vi "Dakota_6Valves.vi"(3 "C/AO0":i32(knob)=472 min=0 max=1023 scale=0.0..1023.0 scale format="%.2f") -> ()   [LabVIEW 2015]
uses:
  <vilib>/rvi/Emulation/niFpgaGetClockAttributes.vi
  <vilib>/rvi/Emulation/niFpgaSctlEmulationGetInTimedLoop.vi
  <vilib>/rvi/Emulation/niFpgaEmulationReportErrorSimple.vi
  <vilib>/rvi/eio/common/nirviEmuTemplateMethod_errors.vi
  <vilib>/rvi/interface/RandomDataEmulation/niFpgaRandomDataHandleErrors.vi
  <vilib>/rvi/Emulation/niFpgaCriticalErrorInLSC.vi
  <vilib>/eio/EIONode/EIONode.xnode
  <vilib>/rvi/DataTransferAndStorage/Container/XNode/niFpgaContainer.xnode
  <vilib>/rvi/interface/RandomDataEmulation/nirviRandomDataFpgaReadWriteTemplate.vi
panel:
  in  "Inlet Count(uSec) 5":i32 caption="Count(uSec)"
  out "A/AO0 Overflow?":bool
  in  "A/AO0":i32(knob)=472 min=0 max=4095 scale=0.0..4095.0 scale format="%.2f"
  in  "Inlet Count(uSec) 4":i32 caption="Count(uSec)"
  out "A/AO1 Overflow?":bool
  in  "A/AO1":i32(knob)=472 min=0 max=4095 scale=0.0..4095.0 scale format="%.2f"
  in  "Inlet Count(uSec) 3":i32 caption="Count(uSec)"
  out "B/AO0 Overflow?":bool
  in  "B/AO0":i32(knob)=472 min=0 max=4095 scale=0.0..4095.0 scale format="%.2f"
  in  "Inlet Count(uSec) 2":i32 caption="Count(uSec)"
  out "B/AO1 Overflow?":bool
  in  "B/AO1":i32(knob)=472 min=0 max=4095 scale=0.0..4095.0 scale format="%.2f"
  in  "Outlet Count(uSec)":i32 caption="Count(uSec)"
  out "C/AO1 Overflow?":bool
  in  "C/AO1":i32(knob)=405 min=0 max=1023 scale=0.0..1023.0 scale format="%.2f"
  in  "Inlet Count(uSec)":i32 caption="Count(uSec)"
  out "C/AO0 Overflow?":bool
  # "Overview\n======\n\nThis demonstrates how to control the PSV105 Valve. At 0 bits, the voltage across the 250 ohms, 30W resistor is 1.3V. This corresponds to 5.2mA, a little above the required current to turn the valve on according to the manufacturer. At 910 bits, we obtain a voltage of 5V across the shunt resistor; this corresponds to 20mA. \n\nConnection Protocols\n===============\nWire the AO0 pin on the C connector of the myRIo to the pin 3 of the non-inverting input of the opamp. Connect the power supplies andfollow the following instructions:\n\nInstructions:\n1.        Operate at constant pressure of 30 psi to get best results\n2.        Operate this valve between the DAC resolutions of 0 and  717 only. If you operate outside of this range, you might damage the valve.\n3.        Run the VI."
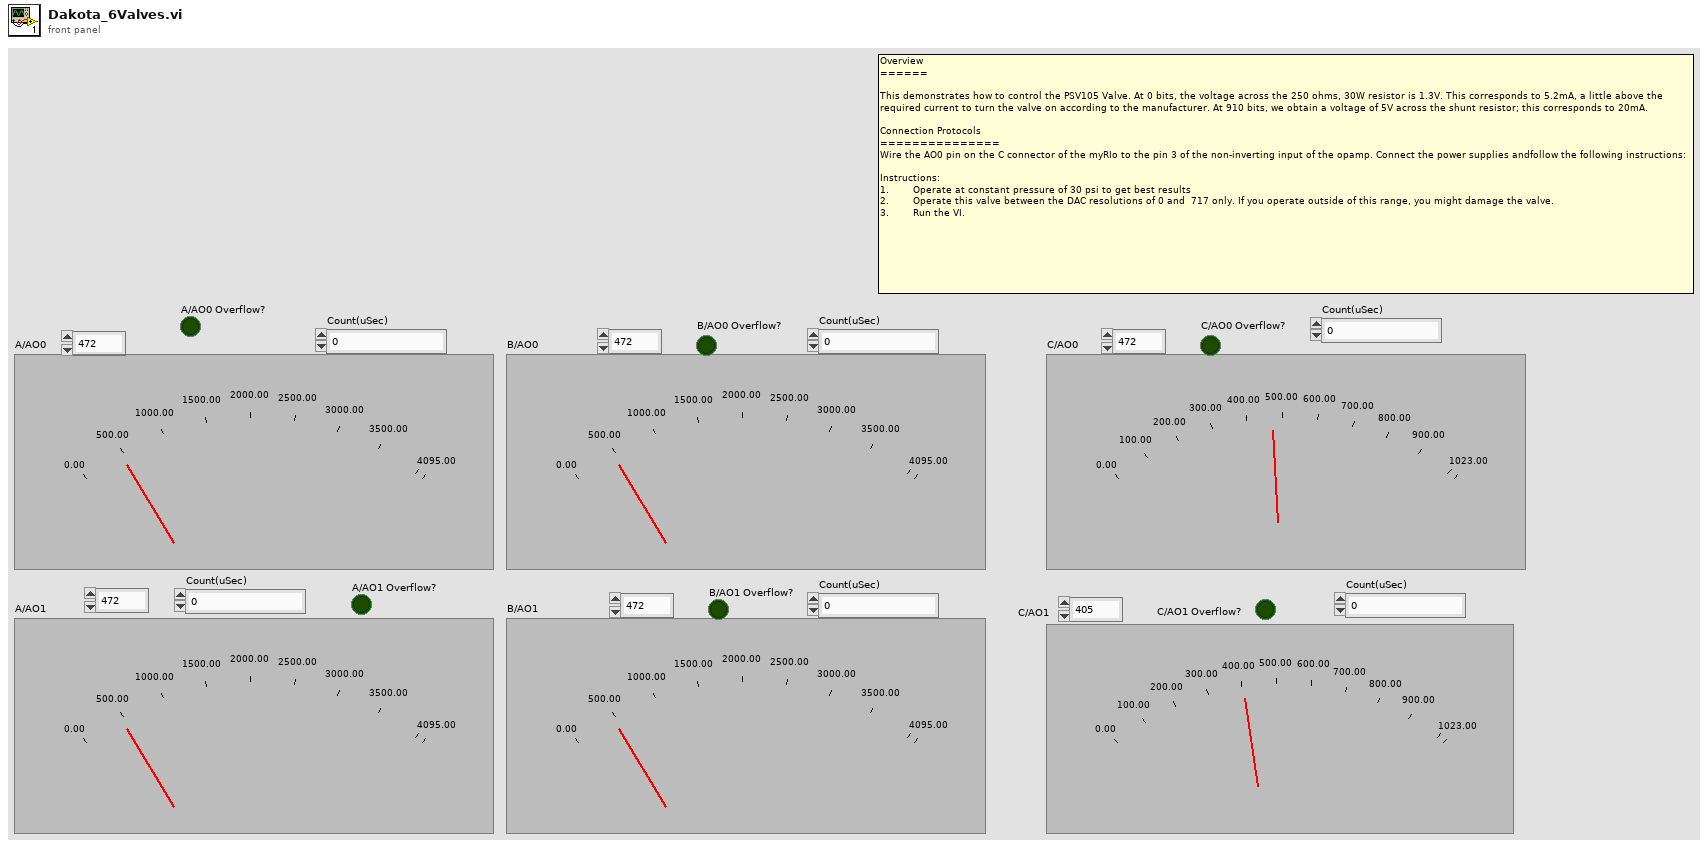
[diagram p1: front panel]
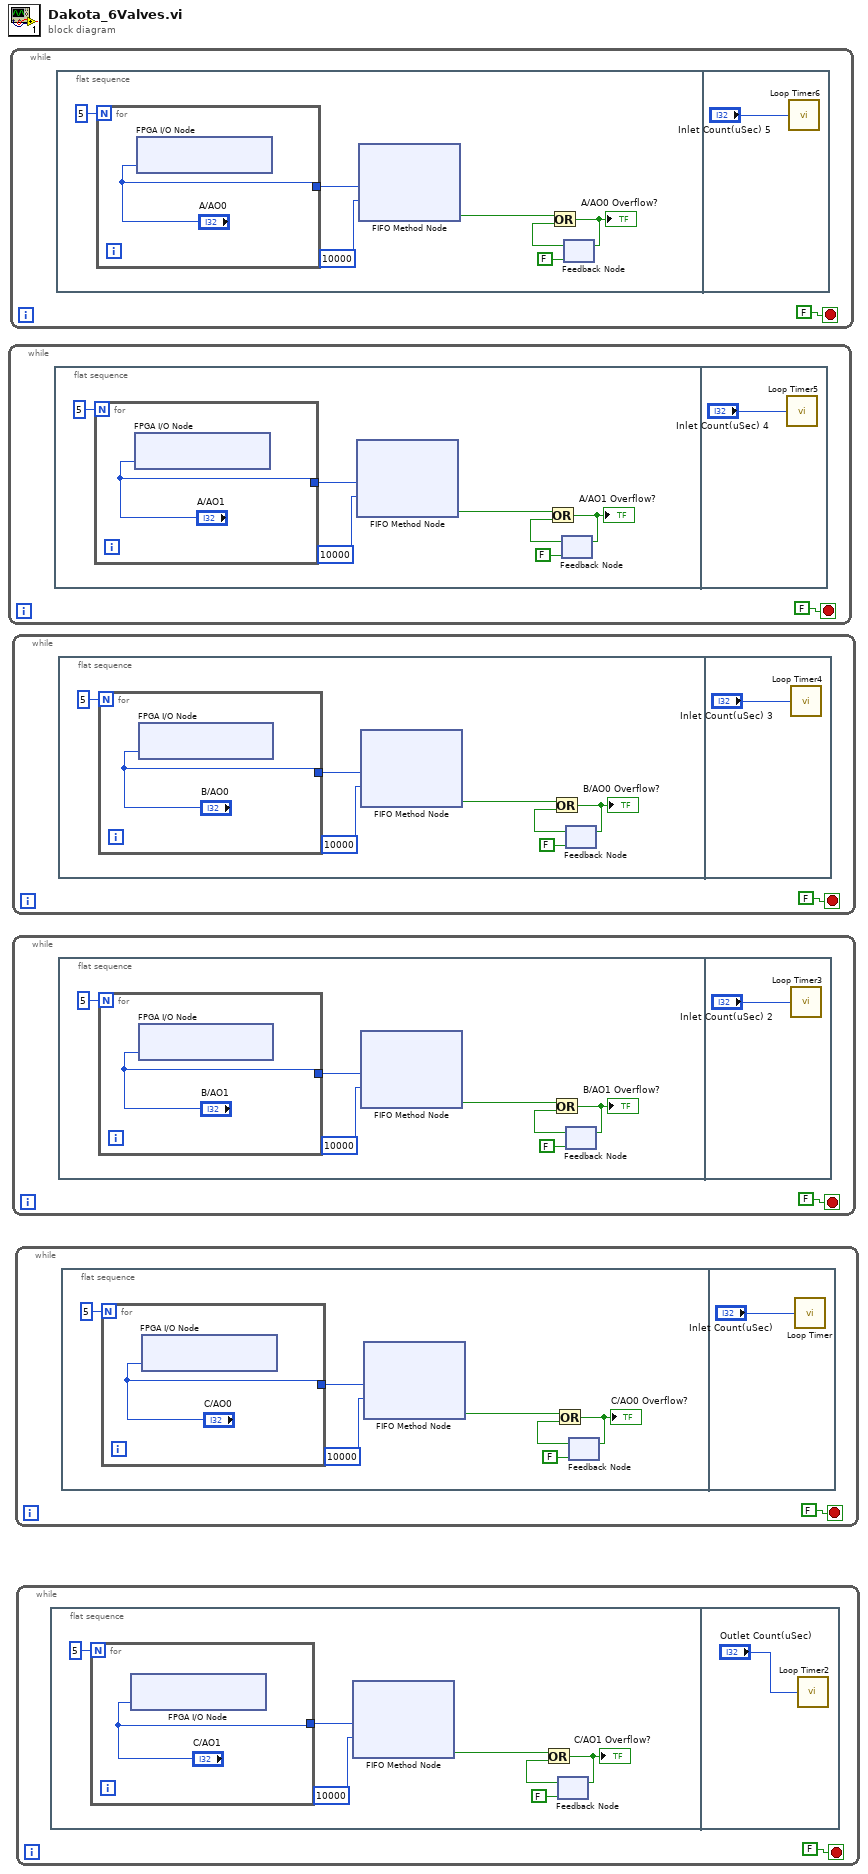
[diagram p0: block diagram]
diagram:
  n1 = while {
    stop <- FALSE stop-if-true
    n2 = flat-sequence {
      frame #0 {
        n3 = for {
          N: 5 -> [_]
          tunnel: ["A/AO1"] -> w3
          n4 = xnode "FPGA I/O Node"("ConnectorA/AO1"="A/AO1") -> ()  [unwired: 1 in, 1 out]
        }
        n5 = xnode ("FIFO Method Node")("Element"=w3, "Timeout"=10000) -> ("Timed Out?"=w5:bool)  [unwired: 1 in, 1 out]
        n6 = feedback #1(FALSE) -> (w7:bool)
        n7 = Or(x=w5, y=w7) -> (x .or. y?=w8:bool)
        "A/AO1 Overflow?" <- w8
        n8 = feedback-in #1(w8) -> ()
      }
      frame #1 {
        n9 = call "Loop Timer5"("Count(uSec)"="Inlet Count(uSec) 4") -> ()  [unwired: 1 out]
      }
    }
  }
  n10 = while {
    stop <- FALSE stop-if-true
    n11 = flat-sequence {
      frame #0 {
        n12 = for {
          N: 5 -> [_]
          tunnel: ["A/AO0"] -> w13
          n13 = xnode "FPGA I/O Node"("ConnectorA/AO0"="A/AO0") -> ()  [unwired: 1 in, 1 out]
        }
        n14 = xnode ("FIFO Method Node")("Element"=w13, "Timeout"=10000) -> ("Timed Out?"=w15:bool)  [unwired: 1 in, 1 out]
        n15 = feedback #2(FALSE) -> (w17:bool)
        n16 = Or(x=w15, y=w17) -> (x .or. y?=w18:bool)
        "A/AO0 Overflow?" <- w18
        n17 = feedback-in #2(w18) -> ()
      }
      frame #1 {
        n18 = call "Loop Timer6"("Count(uSec)"="Inlet Count(uSec) 5") -> ()  [unwired: 1 out]
      }
    }
  }
  n19 = while {
    stop <- FALSE stop-if-true
    n20 = flat-sequence {
      frame #0 {
        n21 = for {
          N: 5 -> [_]
          tunnel: ["B/AO0"] -> w23
          n22 = xnode "FPGA I/O Node"("ConnectorB/AO0"="B/AO0") -> ()  [unwired: 1 in, 1 out]
        }
        n23 = xnode ("FIFO Method Node")("Element"=w23, "Timeout"=10000) -> ("Timed Out?"=w25:bool)  [unwired: 1 in, 1 out]
        n24 = feedback #3(FALSE) -> (w27:bool)
        n25 = Or(x=w25, y=w27) -> (x .or. y?=w28:bool)
        "B/AO0 Overflow?" <- w28
        n26 = feedback-in #3(w28) -> ()
      }
      frame #1 {
        n27 = call "Loop Timer4"("Count(uSec)"="Inlet Count(uSec) 3") -> ()  [unwired: 1 out]
      }
    }
  }
  n28 = while {
    stop <- FALSE stop-if-true
    n29 = flat-sequence {
      frame #0 {
        n30 = for {
          N: 5 -> [_]
          tunnel: ["B/AO1"] -> w33
          n31 = xnode "FPGA I/O Node"("ConnectorB/AO1"="B/AO1") -> ()  [unwired: 1 in, 1 out]
        }
        n32 = xnode ("FIFO Method Node")("Element"=w33, "Timeout"=10000) -> ("Timed Out?"=w35:bool)  [unwired: 1 in, 1 out]
        n33 = feedback #4(FALSE) -> (w37:bool)
        n34 = Or(x=w35, y=w37) -> (x .or. y?=w38:bool)
        "B/AO1 Overflow?" <- w38
        n35 = feedback-in #4(w38) -> ()
      }
      frame #1 {
        n36 = call "Loop Timer3"("Count(uSec)"="Inlet Count(uSec) 2") -> ()  [unwired: 1 out]
      }
    }
  }
  n37 = while {
    stop <- FALSE stop-if-true
    n38 = flat-sequence {
      frame #0 {
        n39 = for {
          N: 5 -> [_]
          tunnel: ["C/AO0"] -> w43
          n40 = xnode "FPGA I/O Node"("ConnectorC/AO0"="C/AO0") -> ()  [unwired: 1 in, 1 out]
        }
        n41 = xnode ("FIFO Method Node")("Element"=w43, "Timeout"=10000) -> ("Timed Out?"=w45:bool)  [unwired: 1 in, 1 out]
        n42 = feedback #5(FALSE) -> (w47:bool)
        n43 = Or(x=w45, y=w47) -> (x .or. y?=w48:bool)
        "C/AO0 Overflow?" <- w48
        n44 = feedback-in #5(w48) -> ()
      }
      frame #1 {
        n45 = call "Loop Timer"("Count(uSec)"="Inlet Count(uSec)") -> ()  [unwired: 1 out]
      }
    }
  }
  n46 = while {
    stop <- FALSE stop-if-true
    n47 = flat-sequence {
      frame #0 {
        n48 = for {
          N: 5 -> [_]
          tunnel: ["C/AO1"] -> w53
          n49 = xnode "FPGA I/O Node"("ConnectorC/AO1"="C/AO1") -> ()  [unwired: 1 in, 1 out]
        }
        n50 = xnode ("FIFO Method Node")("Element"=w53, "Timeout"=10000) -> ("Timed Out?"=w55:bool)  [unwired: 1 in, 1 out]
        n51 = feedback #6(FALSE) -> (w57:bool)
        n52 = Or(x=w55, y=w57) -> (x .or. y?=w58:bool)
        "C/AO1 Overflow?" <- w58
        n53 = feedback-in #6(w58) -> ()
      }
      frame #1 {
        n54 = call "Loop Timer2"("Count(uSec)"="Outlet Count(uSec)") -> ()  [unwired: 1 out]
      }
    }
  }
